vi "Set Guard.vi"(5 "Channel":i32=1 min=1 max=2 step=1, 6 "Channel Guard Status":bool, 7 "Slave":i32=1 min=1 max=6 step=1, 8 "error in (no error)":errorcluster, 11 "VISA resource name":refnum<visa-resource-name>) -> (0 "error out":errorcluster, 3 "VISA resource name out":refnum<visa-resource-name>)   [LabVIEW 2020, in "QuPMXdriver.lvlib"]
doc: "Enable/disable channel guard."
uses:
  QuPMXdriver.lvlib
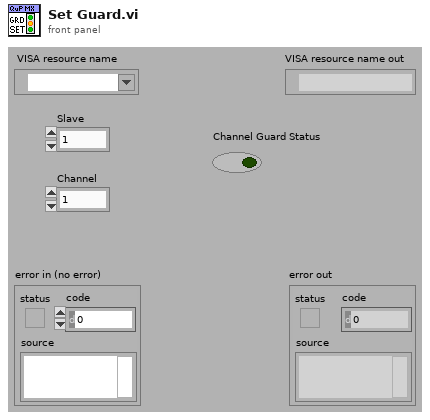
[diagram p1: front panel]
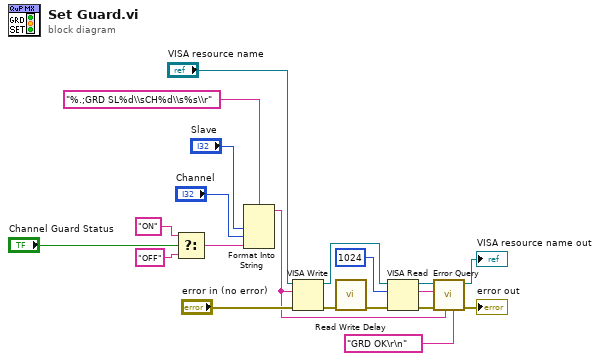
[diagram p0: block diagram]
diagram:
  n1 = Select(t="ON" ("format string"), s="Channel Guard Status", f="OFF" ("format string")) -> (s? t:f=w2:string)
  n2 = Format Into String(format string="%.;GRD SL%d\\sCH%d\\s%s\\r", "Slave", "Channel", w2) -> (resulting string=w8:string)  [unwired: 2 in, 1 out]
  n3 = VISA Write(VISA resource name="VISA resource name", write buffer=w8, error in (no error)="error in (no error)") -> (VISA resource name out=w11:refnum<visa-resource-name>, error out=w15:errorcluster)  [unwired: 1 out]
  n4 = call "Read Write Delay.vi"("error in"=w15) -> ("error out"=w14:errorcluster)  [unwired: 10 in]
  n5 = VISA Read(VISA resource name=w11, byte count=u32 1024, error in (no error)=w14) -> (VISA resource name out=w12:refnum<visa-resource-name>, read buffer=w10:string, error out=w9:errorcluster)  [unwired: 1 out]
  n6 = call "Error Query.vi"("Expected read buffer"="GRD OK\r\n" ("read buffer"), "Last command"=w8, "error in (no error)"=w9, "Read buffer"=w10, "VISA resource name"=w12) -> ("error out"=→"error out":errorcluster, "VISA resource name out"=→"VISA resource name out":refnum<visa-resource-name>)  [unwired: 5 in]
